vi "Protection_debugger.vi"(4 "Transfer Trip":bool, 5 "RMS minimum\nvalues":cluster{"VRMS values":dbl, "IRMS values":dbl}, 6 "Blocking in":bool, 7 "Reset Relay":bool, 8 "input cluster":T3, 9 "Total power values":dbl[](array[numeric]), 10 "RMS values":dbl[](array[numeric]), 11 "Protection settings":T4) -> (0 "output cluster":T3, 1 "Blocking out":bool[](array[boolean]), 2 "Reclose":bool, 3 "trip signal":bool)   [LabVIEW 2016]
uses:
  <vilib>/addons/Electrical Power/Protection/Definite Time Delay/subVIs/fpga_Timer Feedback Var.ctl
  <vilib>/addons/Electrical Power/Protection/Definite Time Delay/subVIs/fpga_State.ctl
  <vilib>/addons/Electrical Power/Protection/Inverse Time Delay/subVIs/ep_Operate Time.ctl
  <vilib>/addons/Electrical Power/Protection/NI_EP_Protection.lvlib
  <vilib>/addons/Electrical Power/Protection/NI_EP_Protection_FPGA.lvlib
panel:
  out "VL error":i32
  out "VR error":i32
  out "I error":i32
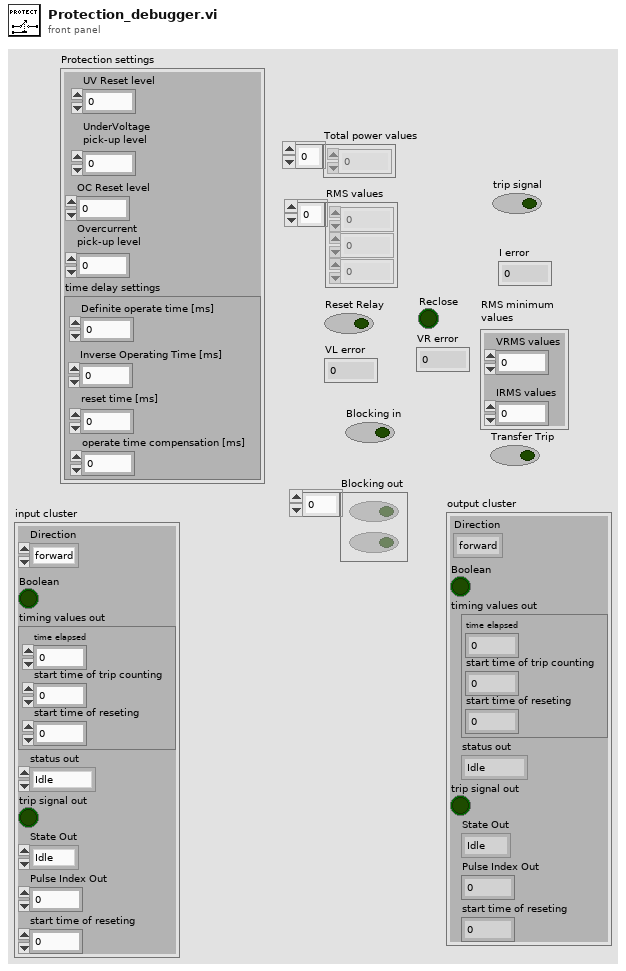
[diagram p1: front panel]
types:
  T1 = typedef "NI_EP_Protection_FPGA.lvlib/fpga_Timer Feedback Var.ctl" = cluster{"time elapsed":u32, "start time of trip counting":u32, "start time of reseting":u32}
  T2 = typedef "NI_EP_Protection_FPGA.lvlib/fpga_State.ctl" = enum16{"Idle", "Trip Counting", "Tripped", "Reset Counting"}
  T3 = cluster{"Direction":enum16{"forward", "backward", "N/D"}, "Boolean":bool, "timing values out":T1, "status out":T2, "trip signal out":bool, "State Out":enum16{"Idle", "Wait for Trip", "PulseClosing", "Locked"}, "Pulse Index Out":i32, "start time of reseting":u32}
  T4 = cluster{"UV Reset level":dbl, "UnderVoltage \npick-up level":dbl, "OC Reset level":dbl, "Overcurrent\npick-up level":dbl, "time delay settings":cluster{"Definite operate time [ms]":u32, "Inverse Operating Time [ms]":u32, "reset time [ms]":u32, "operate time compensation [ms]":u32}}
  T5 = enum16{"Idle", "Wait for Trip", "PulseClosing", "Locked"}
  T6 = cluster{"Definite operate time [ms]":u32, "Inverse Operating Time [ms]":u32, "reset time [ms]":u32, "operate time compensation [ms]":u32}
  T7 = typedef "NI_EP_Protection.lvlib/ep_Operate Time.ctl" = cluster{"A [s]":dbl, "B [s]":dbl, "alpha":dbl, "K2 [s]":dbl, "K1 [s]":dbl, "K3 [s]":dbl}
  T8 = cluster{u32, "reset time [ms]":u32, "reset time [ms]":u32}
  T9 = cluster{"Definite operate time [ms]":u32, "reset time [ms]":u32, "reset time [ms]":u32}
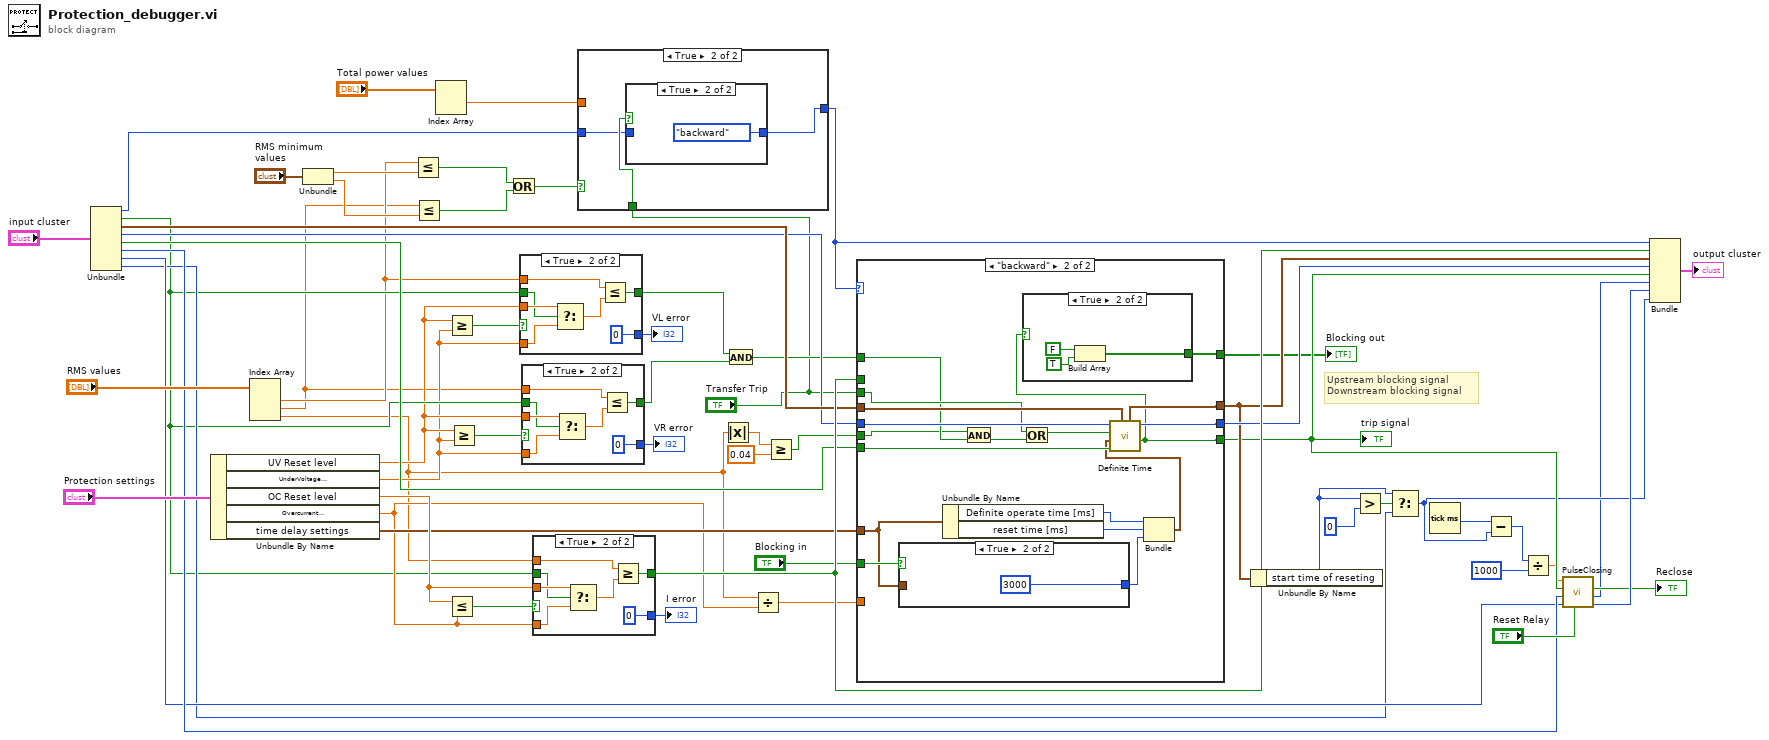
[diagram p0: block diagram]
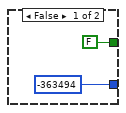
[diagram p2: hidden frame]
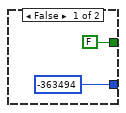
[diagram p3: hidden frame]
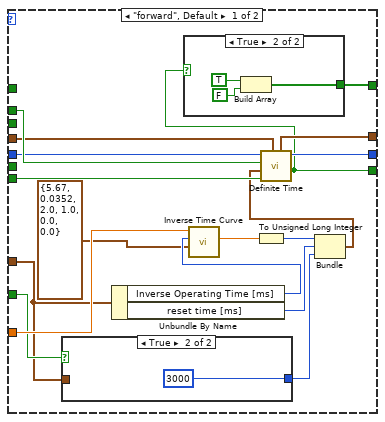
[diagram p4: hidden frame]
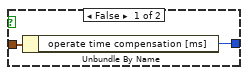
[diagram p5: hidden frame]
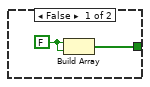
[diagram p6: hidden frame]
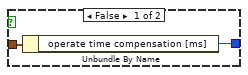
[diagram p7: hidden frame]
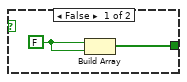
[diagram p8: hidden frame]
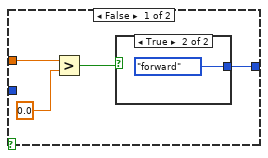
[diagram p9: hidden frame]
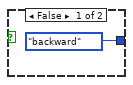
[diagram p10: hidden frame]
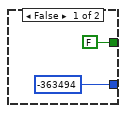
[diagram p12: hidden frame]
diagram:
  # "Upstream blocking signal\nDownstream blocking signal"
  n1 = Unbundle("input cluster") -> ("Direction"=w35:enum16{"forward", "backward", "N/D"}, "Boolean"=w13:bool, "timing values out"=w19:T1, "status out"=w18:T2, "trip signal out"=w17:bool, "State Out"=w16:T5, "Pulse Index Out"=w15:i32, "start time of reseting"=w14:u32)
  n2 = Unbundle By Name("Protection settings") -> ("UV Reset level"=w12:dbl, "UnderVoltage \npick-up level"=w11:dbl, "OC Reset level"=w53:dbl, "Overcurrent\npick-up level"=w38:dbl, "time delay settings"=w51:T6)
  n3 = Index Array(array="RMS values") -> (element #1=w10:dbl, element #2=w9:dbl, element #3=w6:dbl)  [unwired: 3 in]
  n4 = Unbundle("RMS minimum\nvalues") -> ("VRMS values"=w58:dbl, "IRMS values"=w55:dbl)
  n5 = Less Or Equal?(x=w10, y=w58) -> (x <= y?=w57:bool)
  n6 = Less Or Equal?(x=w9, y=w55) -> (x <= y?=w56:bool)
  n7 = Index Array(array="Total power values") -> (element #1=w43:dbl)  [unwired: 2 in, 1 out]
  n8 = Greater Or Equal?(x=w12, y=w11) -> (x >= y?=w22:bool)
  n9 = Less Or Equal?(x=w53, y=w38) -> (x <= y?=w61:bool)
  n10 = Greater Or Equal?(x=w12, y=w11) -> (x >= y?=w24:bool)
  n11 = Or(x=w57, y=w56) -> (x .or. y?=w48:bool)
  n12 = case shown="True" w22 {
    tunnel: [-363494 ("error") 0 ("error")] -> w21
    tunnel: w12 -> [_ w68]
    tunnel: w11 -> [_ w67]
    tunnel: [FALSE ("Boolean") w66] -> w8
    tunnel: w13 -> [_ w65]
    tunnel: w10 -> [_ w64]
    frame False {
    }
    frame True {
      n13 = Select(t=w68, s=w65, f=w67) -> (s? t:f=w70:dbl)
      n14 = Less Or Equal?(x=w64, y=w70) -> (x <= y?=w66:bool)
    }
  }
  "VL error" <- w21
  n15 = case shown="True" w24 {
    tunnel: [-363494 ("error") 0 ("error")] -> w23
    tunnel: w12 -> [_ w77]
    tunnel: w11 -> [_ w76]
    tunnel: [FALSE ("Boolean") w75] -> w7
    tunnel: w13 -> [_ w74]
    tunnel: w9 -> [_ w73]
    frame False {
    }
    frame True {
      n16 = Select(t=w77, s=w74, f=w76) -> (s? t:f=w79:dbl)
      n17 = Less Or Equal?(x=w73, y=w79) -> (x <= y?=w75:bool)
    }
  }
  "VR error" <- w23
  n18 = case shown="True" w61 {
    tunnel: [-363494 ("error") 0 ("error")] -> w60
    tunnel: w53 -> [_ w86]
    tunnel: w38 -> [_ w85]
    tunnel: [FALSE ("Boolean") w84] -> w52
    tunnel: w13 -> [_ w83]
    tunnel: w6 -> [_ w82]
    frame False {
    }
    frame True {
      n19 = Select(t=w86, s=w83, f=w85) -> (s? t:f=w88:dbl)
      n20 = Greater Or Equal?(x=w82, y=w88) -> (x >= y?=w84:bool)
    }
  }
  "I error" <- w60
  n21 = case shown="True" w48 {
    tunnel: w43 -> [w90 _]
    tunnel: w35 -> [_ w95]
    tunnel: [w89 w96] -> w34
    tunnel: "Transfer Trip" -> [_ w97]
    frame False {
      n22 = Greater?(x=w90, y=0.0) -> (0:w91:bool)
      n23 = case shown="True" w91 {
        tunnel: [enum16{"forward", "backward"}."backward" enum16{"forward", "backward"}."forward"] -> w89
        frame False {
        }
        frame True {
        }
      }
    }
    frame True {
      n24 = case shown="True" w97 {
        tunnel: [w98 enum16{"forward", "backward", "N/D"}."backward" ("Direction")] -> w96
        tunnel: w95 -> [w98 _]
        frame False {
        }
        frame True {
        }
      }
    }
  }
  n25 = Absolute Value(x=w6) -> (abs(x)=w1:dbl)
  n26 = And(x=w8, y=w7) -> (x .and. y?=w4:bool)
  n27 = Divide(x=w6, y=w38) -> (x/y=w49:dbl)
  n28 = Greater Or Equal?(x=w1, y=0.04) -> (x >= y?=w3:bool)
  n29 = case shown="\"backward\"" w34 {
    tunnel: w52 -> [w117 _]
    tunnel: w51 -> [w101 w133]
    tunnel: [w116 w138] -> w50
    tunnel: w49 -> [w115 _]
    tunnel: [w114 w139] -> w47
    tunnel: [w113 w137] -> w39
    tunnel: w19 -> [w112 w142]
    tunnel: w18 -> [w111 w141]
    tunnel: w17 -> [w110 w140]
    tunnel: [w103 w136] -> w26
    tunnel: "Blocking in" -> [w102 w135]
    tunnel: w3 -> [_ w126]
    tunnel: w4 -> [_ w128]
    tunnel: "Transfer Trip" -> [_ w129]
    frame "forward", Default {
      n30 = case shown="True" w102 {
        tunnel: [w118 u32 3000 ("reset time [ms]")] -> w100
        tunnel: w101 -> [w119 _]
        frame False {
          n31 = Unbundle By Name(w119) -> ("operate time compensation [ms]"=w118:u32)
        }
        frame True {
        }
      }
      n32 = Unbundle By Name(w101) -> ("Inverse Operating Time [ms]"=w109:u32, "reset time [ms]"=w106:u32)
      n33 = call "Inverse Time Curve.vi"("input cluster"=T7 {"A [s]"=5.67, "B [s]"=0.0352, "alpha"=2.0, "K2 [s]"=1.0, "K1 [s]"=0.0, "K3 [s]"=0.0}, "time dial"=w109, "multiples of pickup"=w115) -> ("original time"=w107:dbl)  [unwired: 5 in, 1 out]
      n34 = To Unsigned Long Integer(number=w107) -> (unsigned 32bit integer=w104:u32)
      n35 = Bundle(w104, "reset time [ms]"=w106, "reset time [ms]"=w100) -> (w105:T8)  [unwired: 1 in]
      n36 = call "Definite Time.vi"("timing values in"=w112, "trip signal in"=w110, "time delay settings"=w105, "pick-up signal? (F)"=w117, "status in"=w111) -> ("trip signal out"=w113:bool, "status out"=w116:T2, "timing values out"=w114:T1)  [unwired: 3 in, 1 out]
      n37 = case shown="True" w113 {
        tunnel: [w121 w123] -> w103
        frame False {
          w122 = FALSE
          n38 = Build Array(w122, w122) -> (w121:bool[])
        }
        frame True {
          n39 = Build Array(TRUE, FALSE) -> (w123:bool[])
        }
      }
    }
    frame "backward" {
      n40 = case shown="True" w135 {
        tunnel: [w144 u32 3000 ("reset time [ms]")] -> w134
        tunnel: w133 -> [w145 _]
        frame False {
          n41 = Unbundle By Name(w145) -> ("operate time compensation [ms]"=w144:u32)
        }
        frame True {
        }
      }
      n42 = Unbundle By Name(w133) -> ("Definite operate time [ms]"=w132:u32, "reset time [ms]"=w143:u32)
      n43 = And(x=w126, y=w128) -> (x .and. y?=w127:bool)
      n44 = Or(x=w129, y=w127) -> (x .or. y?=w130:bool)
      n45 = Bundle("Definite operate time [ms]"=w132, "reset time [ms]"=w143, "reset time [ms]"=w134) -> (w131:T9)  [unwired: 1 in]
      n46 = call "Definite Time.vi"("timing values in"=w142, "trip signal in"=w140, "time delay settings"=w131, "pick-up signal? (F)"=w130, "status in"=w141) -> ("trip signal out"=w137:bool, "status out"=w138:T2, "timing values out"=w139:T1)  [unwired: 3 in, 1 out]
      n47 = case shown="True" w137 {
        tunnel: [w147 w149] -> w136
        frame False {
          w148 = FALSE
          n48 = Build Array(w148, w148) -> (w147:bool[])
        }
        frame True {
          n49 = Build Array(FALSE, TRUE) -> (w149:bool[])
        }
      }
    }
  }
  "trip signal" <- w39
  "Blocking out" <- w26
  n50 = Unbundle By Name(w47) -> ("start time of reseting"=w31:u32)
  n51 = Greater?(x=w31, y=u32 0 ("x")) -> (0:w32:bool)
  n52 = Select(t=w31, s=w32, f=w14) -> (s? t:f=w30:u32)
  n53 = Tick Count (ms)() -> (millisecond timer value=w46:u32)
  n54 = Subtract(x=w46, y=w30) -> (x-y=w41:u32)
  n55 = Divide(x=w41, y=u32 1000) -> (x/y=w29:dbl)
  n56 = call "PulseClosing.vi"("Reset Relay"="Reset Relay", "Pulse Index In"=w15, "State In"=w16, "Trip signal"=w39, "Time lapsed"=w29) -> ("Pulse Index Out"=w40:i32, "State Out"=w28:T5, "Reclose"=→"Reclose":bool)  [unwired: 4 in]
  n57 = Bundle("Direction"=w34, "Boolean"=w52, "timing values out"=w47, "status out"=w50, "trip signal out"=w39, "State Out"=w28, "Pulse Index Out"=w40, "start time of reseting"=w30) -> (→"output cluster":T3)  [unwired: 1 in]
